vi "chunk_trace.vi"(4 "After":dbl, 5 "Note":bool[](array[boolean])=[FALSE, FALSE, TRUE, TRUE, FALSE, FALSE, FALSE, FALSE, FALSE, FALSE, FALSE, FALSE, FALSE, FALSE, FALSE, TRUE, TRUE], 6 "Before":dbl, 7 "Flag names":string[](array[string]), 8 "Max len":dbl=120.0, 9 "Condition":T1[](array[typedef])=[enum."*", enum."*", enum."*", enum."*", enum."*", enum."*", enum."*", enum."*", enum."*", enum."*", enum."*", enum."*", enum."*", enum."*", enum."*", enum."*", enum."*"], 11 "Index array":T2[](array[typedef]) {"Timestamp" format="%<%.3X>T"}) -> (2 "Descriptions":string[][](array[string]), 3 "Chunks":cluster{T2[]}[](array[cluster]) {"?"."Timestamp" format="%<%.3X>T"})   [LabVIEW 2012]
uses:
  ltrace_index.ctl
  bool_condition.ctl
panel:
  # "Maximum chunk length (sec)"
  # "Seconds of data before and after the records with the specified condition.   If an invalid gap is less than \"After\", then it does not terminate the chunk."
  # "Condition on the boolean flags in trace index: false, true or any (don't care.)  First two flags are tracing and OCT data, rest are status flags.\n\nNote says whether to report flag in description."
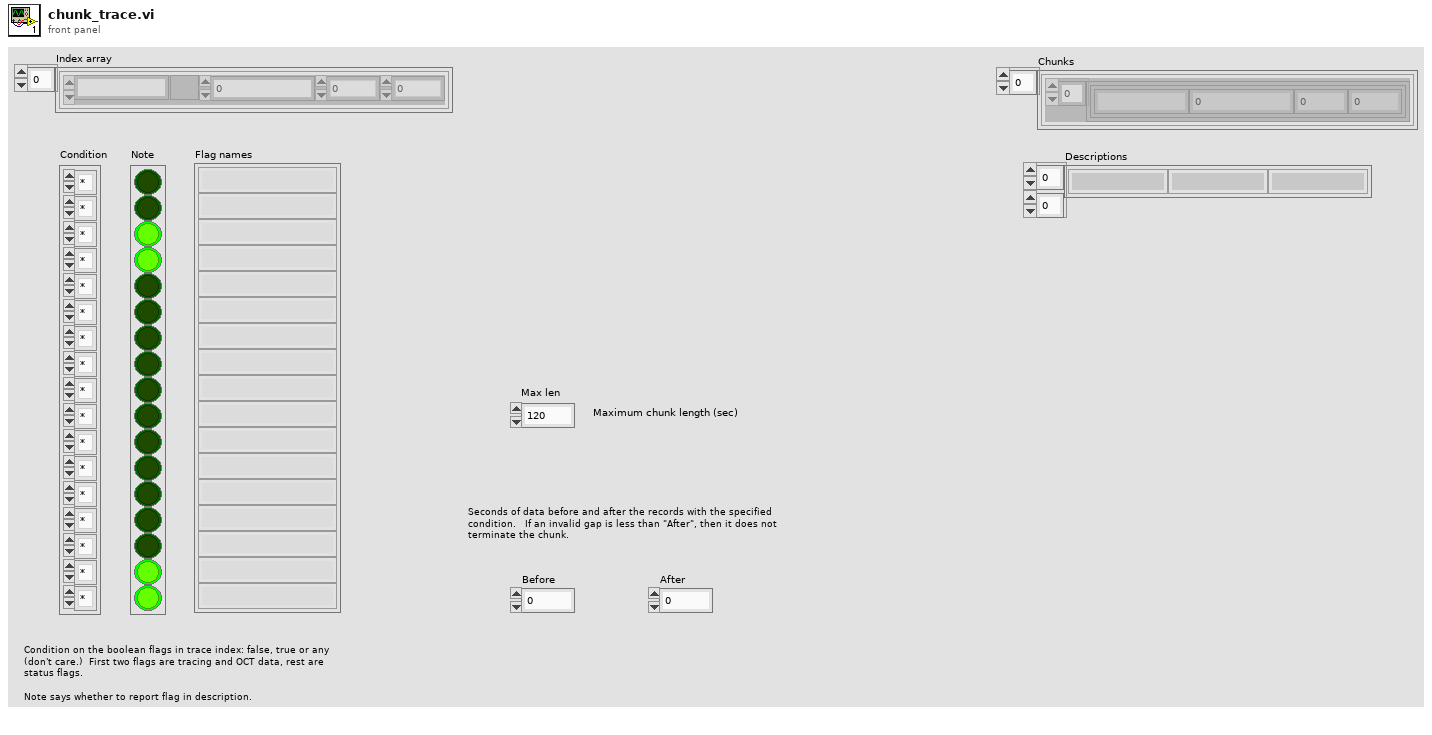
[diagram p1: front panel]
types:
  T1 = typedef "bool_condition.ctl" = enum16{"0", "1", "*"}
  T2 = typedef "ltrace_index.ctl" = cluster{"Timestamp":timestamp, "Offset":i64, "Sequence":u32, "Flags":u32}
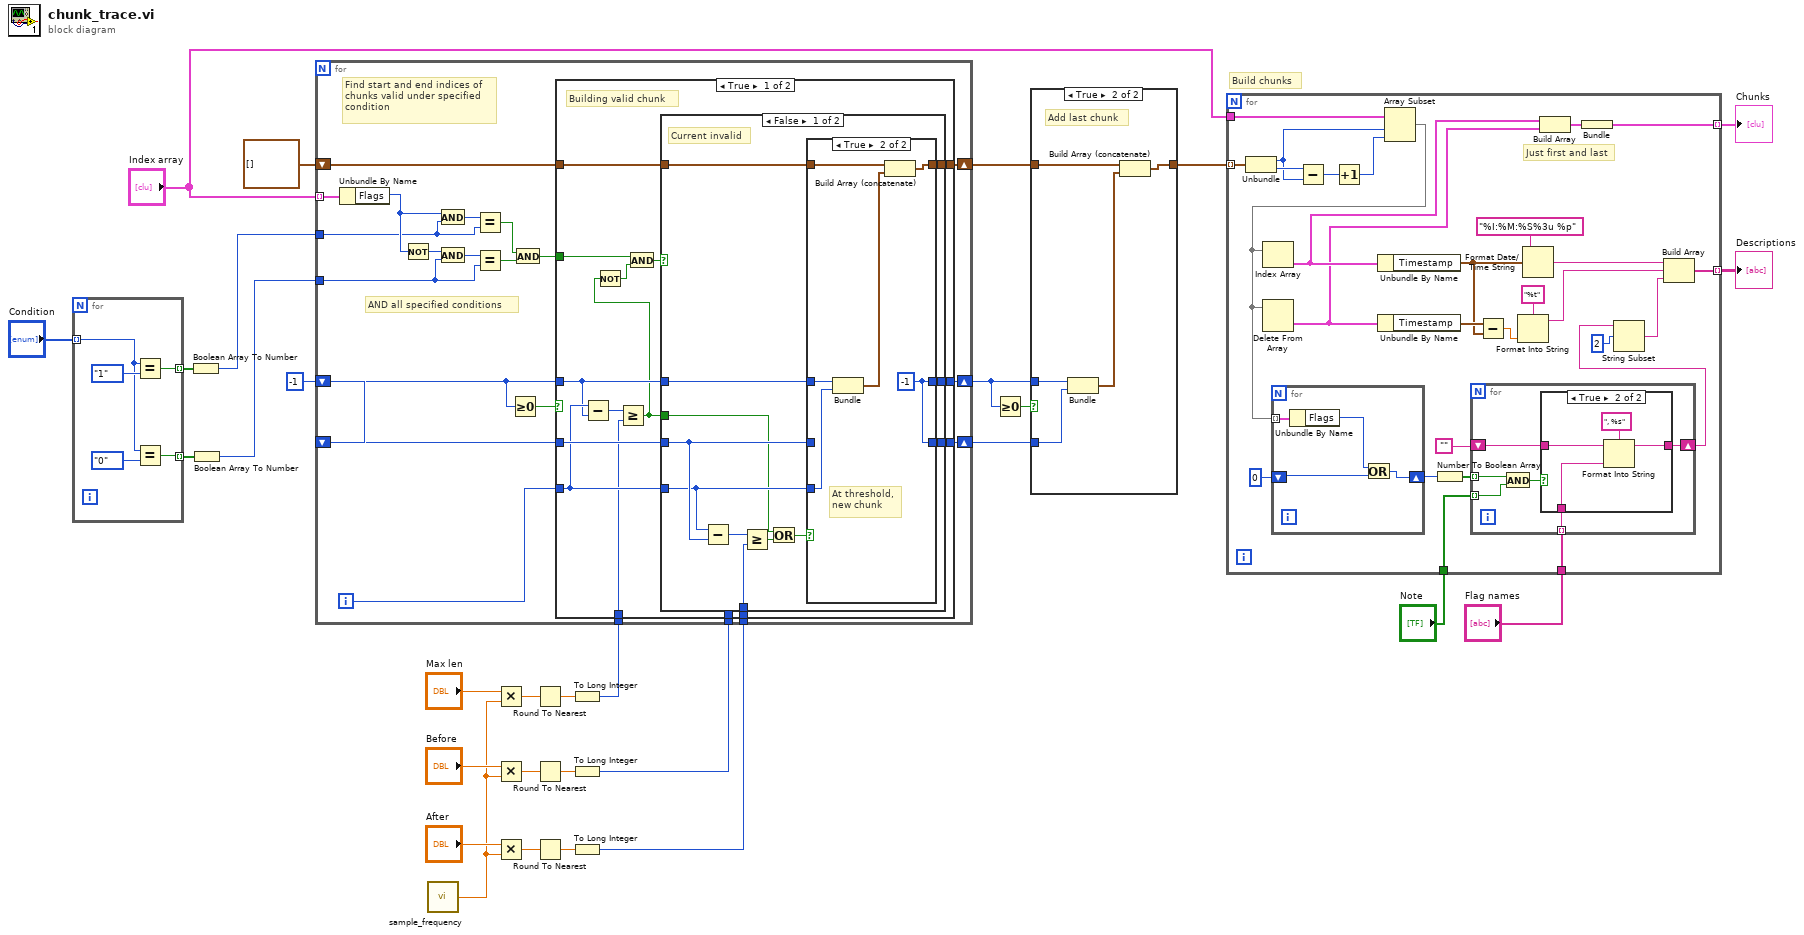
[diagram p0: block diagram]
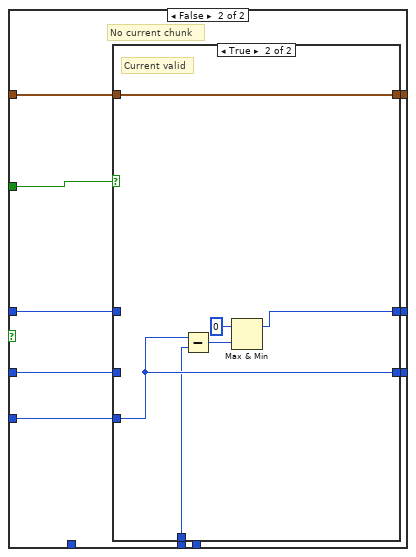
[diagram p6: hidden frame]
diagram:
  w21 = -1 ("output 3")
  # "Build chunks"
  n1 = for {
    tunnel: "Condition" -> [w32] mode=indexing
    tunnel: [w31] -> w9 mode=indexing
    tunnel: [w34] -> w11 mode=indexing
    n2 = Equal?(x=w32, y=bool_condition."1") -> (x = y?=w34:bool)
    n3 = Equal?(x=w32, y=bool_condition."0") -> (x = y?=w31:bool)
  }
  n4 = Boolean Array To Number(Boolean array=w11) -> (number=w10:u32)
  n5 = Boolean Array To Number(Boolean array=w9) -> (number=w8:u32)
  n6 = call "sample_frequency.vi"() -> ("Sample frequency"=w2:dbl)
  n7 = Multiply(x="Max len", y=w2) -> (x*y=w4:dbl)
  n8 = Multiply(x="Before", y=w2) -> (x*y=w17:dbl)
  n9 = Multiply(x="After", y=w2) -> (x*y=w16:dbl)
  n10 = Round To Nearest(number=w4) -> (nearest integer value=w5:dbl)
  n11 = Round To Nearest(number=w17) -> (nearest integer value=w15:dbl)
  n12 = Round To Nearest(number=w16) -> (nearest integer value=w14:dbl)
  n13 = To Long Integer(number=w5) -> (32bit integer=w1:i32)
  n14 = To Long Integer(number=w15) -> (32bit integer=w12:i32)
  n15 = To Long Integer(number=w14) -> (32bit integer=w13:i32)
  n16 = for {
    tunnel: "Index array" -> [w56] mode=indexing
    shift-right: [w51] -> w26
    shift-left: w21 -> [w44]
    shift-right: [w50] -> w27
    shift-left: w21 -> [w54]
    shift-right: [w52] -> w28
    shift-left: cluster{"output 3":i32, "output 3":i32}[] [] -> [w53]
    tunnel: w10 -> [w38]
    tunnel: w13 -> [w49]
    tunnel: w12 -> [w48]
    tunnel: w8 -> [w40]
    tunnel: w1 -> [w42]
    i -> [w45]
    # "AND all specified conditions"
    # "Find start and end indices of\nchunks valid under specified\ncondition"
    n17 = Unbundle By Name(w56) -> ("Flags"=w47:u32)
    n18 = Not(x=w47) -> (.not. x?=w46:u32)
    n19 = And(x=w47, y=w38) -> (x .and. y?=w39:u32)
    n20 = And(x=w46, y=w40) -> (x .and. y?=w41:u32)
    n21 = Equal?(x=w39, y=w38) -> (x = y?=w37:bool)
    n22 = Equal?(x=w41, y=w40) -> (x = y?=w36:bool)
    n23 = Greater Or Equal To 0?(x=w44) -> (x >= 0?=w55:bool)
    n24 = And(x=w37, y=w36) -> (x .and. y?=w43:bool)
    n25 = case shown="True" w55 {
      tunnel: w43 -> [w63 w103]
      tunnel: w44 -> [w60 w102]
      tunnel: w54 -> [w70 w101]
      tunnel: w45 -> [w61 w100]
      tunnel: w53 -> [w69 w99]
      tunnel: [w68 w98] -> w52
      tunnel: [w67 w97] -> w51
      tunnel: [w66 w96] -> w50
      tunnel: w49 -> [w65 _]
      tunnel: w48 -> [_ w95]
      tunnel: w42 -> [w59 _]
      frame True {
        # "Building valid chunk"
        n26 = Subtract(x=w61, y=w60) -> (x-y=w62:i32)
        n27 = Greater Or Equal?(x=w62, y=w59) -> (x >= y?=w58:bool)
        n28 = Not(x=w58) -> (.not. x?=w64:bool)
        n29 = And(x=w63, y=w64) -> (x .and. y?=w57:bool)
        n30 = case shown="False" w57 {
          tunnel: w60 -> [w74 w93]
          tunnel: w70 -> [w76 _]
          tunnel: w61 -> [w75 w92]
          tunnel: w69 -> [w82 w94]
          tunnel: [w79 w94] -> w68
          tunnel: [w81 w93] -> w67
          tunnel: [w80 w92] -> w66
          tunnel: w65 -> [w77 _]
          tunnel: w58 -> [w71 _]
          frame False {
            # "Current invalid"
            n31 = Subtract(x=w75, y=w76) -> (x-y=w78:i32)
            n32 = Greater Or Equal?(x=w78, y=w77) -> (x >= y?=w73:bool)
            n33 = Or(x=w71, y=w73) -> (x .or. y?=w72:bool)
            n34 = case shown="True" w72 {
              tunnel: w74 -> [w84 w91]
              tunnel: w75 -> [_ w90]
              tunnel: w82 -> [w85 w89]
              tunnel: [w85 w87] -> w79
              tunnel: [w84 w86] -> w81
              tunnel: [w83 w86] -> w80
              tunnel: w76 -> [w83 _]
              frame False {
                # "Below threshold"
              }
              frame True {
                w86 = -1 ("output 3")
                # "At threshold,\nnew chunk"
                n35 = Bundle("output 3"=w91, w90) -> (w88:cluster{"output 3":i32, i32})  [unwired: 1 in]
                n36 = Build Array (concatenate)(w89, w88) -> (w87:cluster{"output 3":i32, "output 3":i32}[])
              }
            }
          }
          frame True {
            # "Current valid"
          }
        }
      }
      frame False {
        # "No current chunk"
        n37 = case shown="True" w103 {
          tunnel: w102 -> [w106 _]
          tunnel: w101 -> [w105 _]
          tunnel: w100 -> [_ w111]
          tunnel: w99 -> [w104 w112]
          tunnel: [w104 w112] -> w98
          tunnel: [w106 w107] -> w97
          tunnel: [w105 w111] -> w96
          tunnel: w95 -> [_ w110]
          frame False {
            # "Current invalid"
          }
          frame True {
            # "Current valid"
            n38 = Subtract(x=w111, y=w110) -> (x-y=w109:i32)
            n39 = Max & Min(x=0, y=w109) -> (max(x,y)=w107:i32)  [unwired: 1 out]
          }
        }
      }
    }
  }
  n40 = Greater Or Equal To 0?(x=w26) -> (x >= 0?=w25:bool)
  n41 = case shown="True" w25 {
    tunnel: w26 -> [_ w117]
    tunnel: w27 -> [_ w116]
    tunnel: w28 -> [w113 w115]
    tunnel: [w113 w114] -> w29
    frame False {
    }
    frame True {
      # "Add last chunk"
      n42 = Bundle("output 3"=w117, "output 3"=w116) -> (w118:cluster{"output 3":i32, "output 3":i32})  [unwired: 1 in]
      n43 = Build Array (concatenate)(w115, w118) -> (w114:cluster{"output 3":i32, "output 3":i32}[])
    }
  }
  n44 = for {
    tunnel: w29 -> [w146] mode=indexing
    tunnel: "Index array" -> [w145]
    tunnel: [w142] -> w23 mode=indexing
    tunnel: [w137] -> w24 mode=indexing
    tunnel: "Note" -> [w127]
    tunnel: "Flag names" -> [w126]
    # "Just first and last"
    n45 = Unbundle(w146) -> ("output 3"=w143:i32, "output 3"=w144:i32)
    n46 = Subtract(x=w144, y=w143) -> (x-y=w133:i32)
    n47 = Increment(x=w133) -> (x+1=w132:i32)
    n48 = Array Subset(array=w145, index=w143, length=w132) -> (w131:T2[])
    n49 = Index Array(array=w131) -> (element=w121:T2)  [unwired: 1 in]
    n50 = Delete From Array(array=w131) -> (deleted portion=w120:T2)  [unwired: 2 in, 1 out]
    n51 = for {
      tunnel: w131 -> [w161] mode=indexing
      shift-right: [w158] -> w129
      shift-left: u32 0 ("Flags") -> [w160]
      n52 = Unbundle By Name(w161) -> ("Flags"=w159:u32)
      n53 = Or(x=w159, y=w160) -> (x .or. y?=w158:u32)
    }
    n54 = Unbundle By Name(w121) -> ("Timestamp"=w140:timestamp)
    n55 = Unbundle By Name(w120) -> ("Timestamp"=w141:timestamp)
    n56 = Number To Boolean Array(number=w129) -> (Boolean array=w128:bool[])
    n57 = for {
      tunnel: w128 -> [w152] mode=indexing
      tunnel: w127 -> [w151] mode=indexing
      tunnel: w126 -> [w147] mode=indexing
      shift-right: [w148] -> w124
      shift-left: "" -> [w149]
      n58 = And(x=w152, y=w151) -> (x .and. y?=w150:bool)
      n59 = case shown="True" w150 {
        tunnel: w149 -> [w153 w157]
        tunnel: [w153 w155] -> w148
        tunnel: w147 -> [_ w154]
        frame False {
        }
        frame True {
          n60 = Format Into String(format string=", %s", initial string=w157, w154) -> (resulting string=w155:string)  [unwired: 1 in, 1 out]
        }
      }
    }
    n61 = Subtract(x=w141, y=w140) -> (x-y=w135:dbl)
    n62 = Format Into String(format string="%t" ("time format string (%c)"), w135) -> (resulting string=w134:string)  [unwired: 2 in, 1 out]
    n63 = Format Date/Time String(time format string (%c)="%I:%M:%S%3u %p", seconds (now)=w140) -> (date/time string=w138:string)  [unwired: 1 in]
    n64 = Build Array(w121, w120) -> (w119:T2[])
    n65 = Bundle(w119) -> (w142:cluster{T2[]})  [unwired: 1 in]
    n66 = String Subset(string=w124, offset (0)=2) -> (substring=w123:string)  [unwired: 1 in]
    n67 = Build Array(w138, w134, w123) -> (w137:string[])
  }
  "Chunks" <- w23
  "Descriptions" <- w24
